vi "Scatter Page.vi"() -> ()   [LabVIEW 2020, in "3D Scatter.lvclass"]
uses:
  <vilib>/Math Plots/3D Math Plots/3D Scatter/3D Scatter/3D Scatter.lvclass
  <vilib>/Math Plots/3D Math Plots/3D Scatter/3D Scatter/Typedef/3D Scatter Property Array.ctl
  <vilib>/Math Plots/3D Math Plots/3D Scatter/3D Scatter/Typedef/3D Scatter Property.ctl
  <vilib>/Math Plots/3D Math Plots/3D Plot/3D Plot/Typedef/Sprite Type.ctl
  <vilib>/Math Plots/3D Math Plots/3D Plot/3D Plot/Typedef/Color Ramp Cluster.ctl
  <vilib>/Math Plots/3D Math Plots/3D Plot/3D Plot/Typedef/Dialog State.ctl
  <vilib>/Math Plots/3D Math Plots/3D Plot/3D Plot/Typedef/Temp Scene State.ctl
  <vilib>/Math Plots/3D Math Plots/3D Plot/3D Plot/Typedef/Temp Scene Property Action.ctl
  <vilib>/Math Plots/3D Math Plots/3D Plot/3D Plot/3D Plot.lvclass
panel:
  in  "Point Size":sgl=0.001 caption="Point size" min=0.001 step=1
  in  "Point Style":u16(ring) caption="Point style"
  out "Scatter Property Out":T1
  in  "Scatter Property In":T1
  out "Color Ramp":dbl[][](graph)
  in  "Color Map Style":u16(ring) caption="Color map style" items=["None ", "Shaded", "Color spectrum", "Grey scale", "Custom"]
  in  "YZ Plane Projection":bool caption="YZ plane projection"
  in  "XZ Plane Projection":bool caption="XZ plane projection"
  in  "XY Plane Projection":bool caption="XY plane projection"
  in  "Coordinate System":u16(ring) caption="Coordinate system" items=["Cartesian", "Cylindrical", "Spherical"]
  in  "Plot Opacity":sgl(slide) caption="Plot opacity(%)" min=0 max=100 scale=0.0..100.0
  in  "Plot List":i32(listbox)
  in  "Ramp Edit":bool caption="Ramp edit"
  in  "Move Down":bool
  in  "Move Up":bool
  in  "Delete":bool
  in  "New":bool
  in  "Event Registration":refnum<event-registration>
  # "Scatter"
  # "General"
  # "Projection"
  # "Color Ramp"
  # "Scatter"
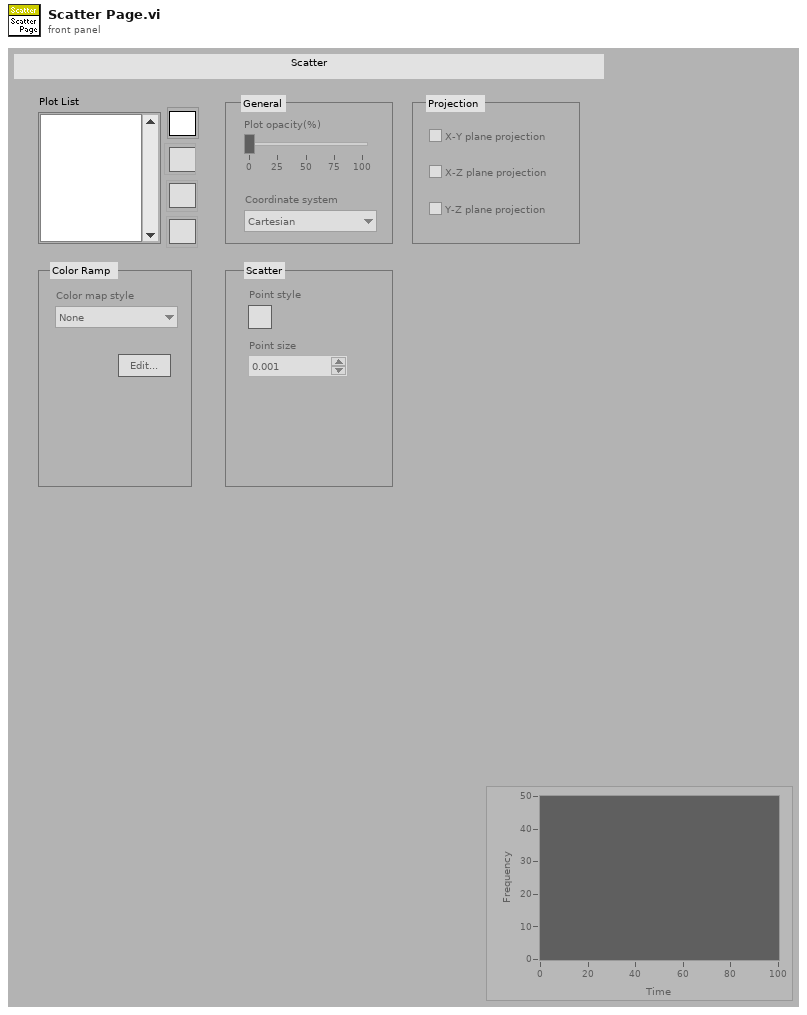
[diagram p1: front panel]
types:
  T1 = typedef "3D Scatter.lvclass/3D Scatter Property Array.ctl" = T2[]
  T2 = typedef "3D Scatter.lvclass/3D Scatter Property.ctl" = cluster{"General Property":cluster{"Plot Name":string, "Coordinate System":enum16{"Cartesian", "Cylindrical", "Spherical"}, "Opacity":sgl}, "Projection Property":cluster{"Draw XY":bool, "Draw YZ":bool, "Draw XZ":bool}, "Plot Property":cluster{"Sprite Type":T3, "Point Size":sgl, "Color Ramp Cluster":T4}}
  T3 = typedef "3D Plot.lvclass/Sprite Type.ctl" = enum16{"None", "Empty Square", "Solid Square", "Empty Diamond", "Solid Diamond", "Empty Circle", "Solid Circle", "Asterisk", "Bold X", "Wireframe Sphere", "Solid Sphere", "Wireframe Cube", "Solid Cube"}
  T4 = typedef "3D Plot.lvclass/Color Ramp Cluster.ctl" = cluster{"Color Ramp Style":enum16{"None", "Shaded", "Color spectrum", "Grey scale", "Custom"}, "Color Ramp Array":u32[], "Color Ramp Index":i32[], "Interpolate?":bool, "Logarithm?":bool}
  T5 = typedef "3D Plot.lvclass/Dialog State.ctl" = enum16{"Initialize", "Read Porperty", "Write Property", "Idle", "Exit"}
  T6 = typedef "3D Plot.lvclass/Temp Scene State.ctl" = enum16{"Create", "Update Scene", "Get Plot Representation", "Destory"}
  T7 = typedef "3D Plot.lvclass/Temp Scene Property Action.ctl" = enum16{"Graph Property", "Light Property", "Axis Property", "Value Pair Property", "Format Property", "Cursor Property", "Plot Specific Property"}
  T8 = typedef "3D Plot.lvclass/Multiplot Representation.ctl" = cluster{"Plot Represention Array":T9[], "Max Range":T10}
  T9 = typedef "3D Plot.lvclass/Plot Representation.ctl" = cluster{"Plot ID":i32, "Plot Range":T10, "Mesh Data":T11, "Dimension":cluster{"X Dimension":i32, "Y Dimension":i32}, "Ramp Range":T10}
  T10 = typedef "3D Plot.lvclass/Range Clusters.ctl" = cluster{"X Range":cluster{"Max X":sgl, "Min X":sgl}, "Y Range":cluster{"Max Y":sgl, "Min Y":sgl}, "Z Range":cluster{"Max Z":sgl, "Min Z":sgl}}
  T11 = typedef "3D Plot.lvclass/Mesh Data.ctl" = cluster{"Index Array":u32[], "Vertex Array":cluster{"X":sgl, "Y":sgl, "Z":sgl}[], "Normal Array":cluster{"X":sgl, "Y":sgl, "Z":sgl}[], "Color Index Array":i32[]}
  T12 = enum16{"None", "Shaded", "Color spectrum", "Grey scale", "Custom"}
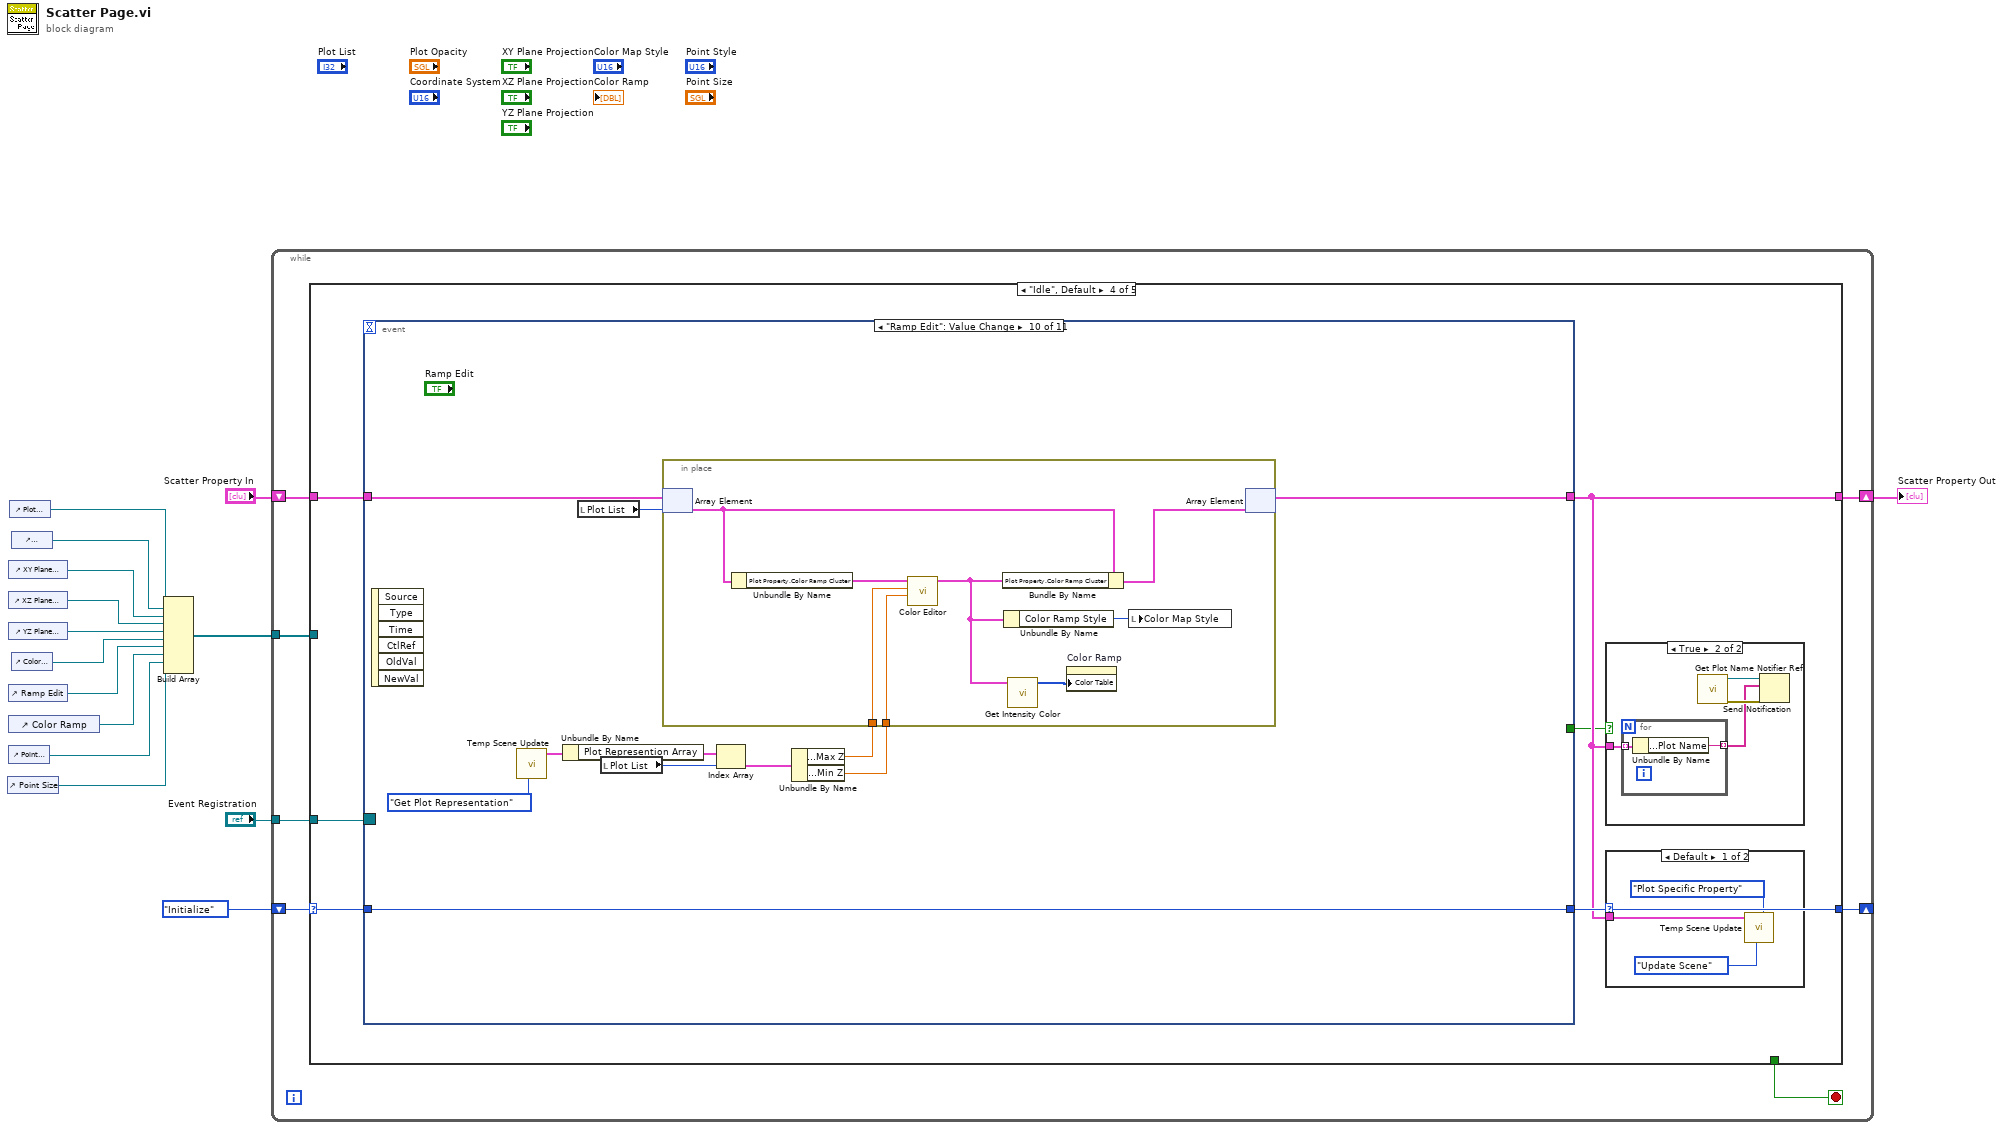
[diagram p0: block diagram]
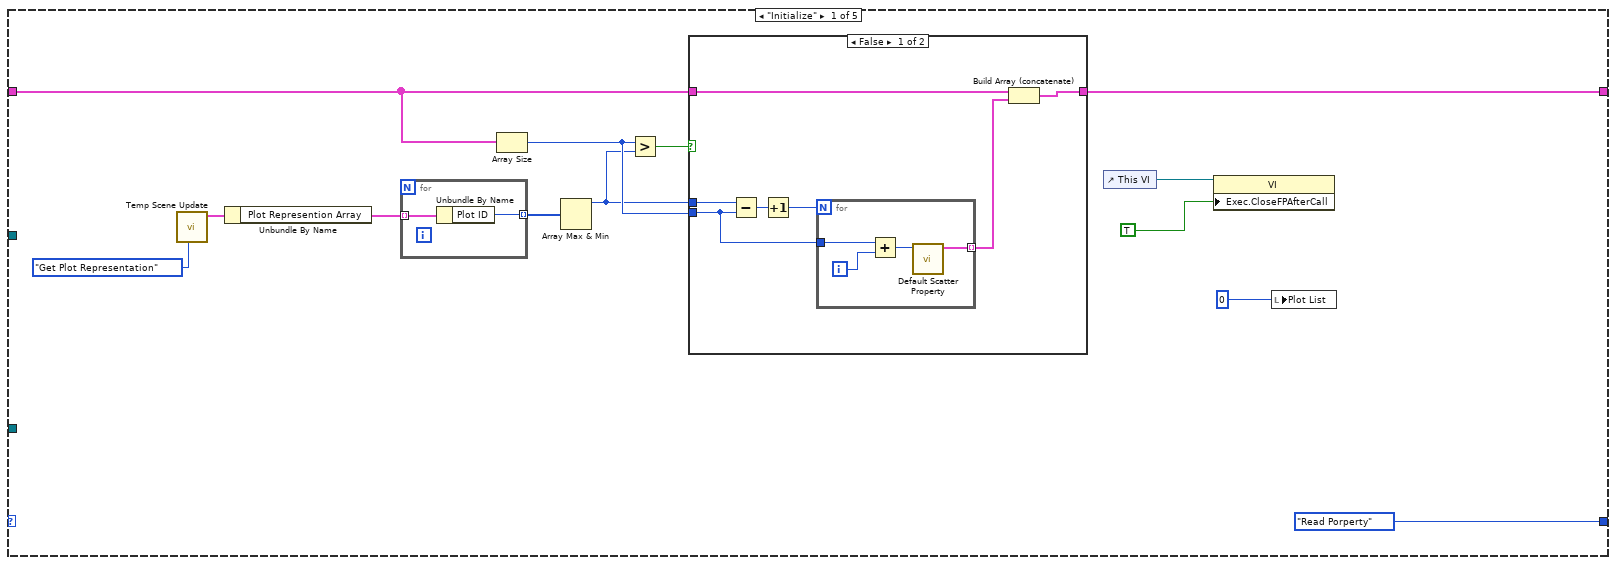
[diagram p2: hidden frame]
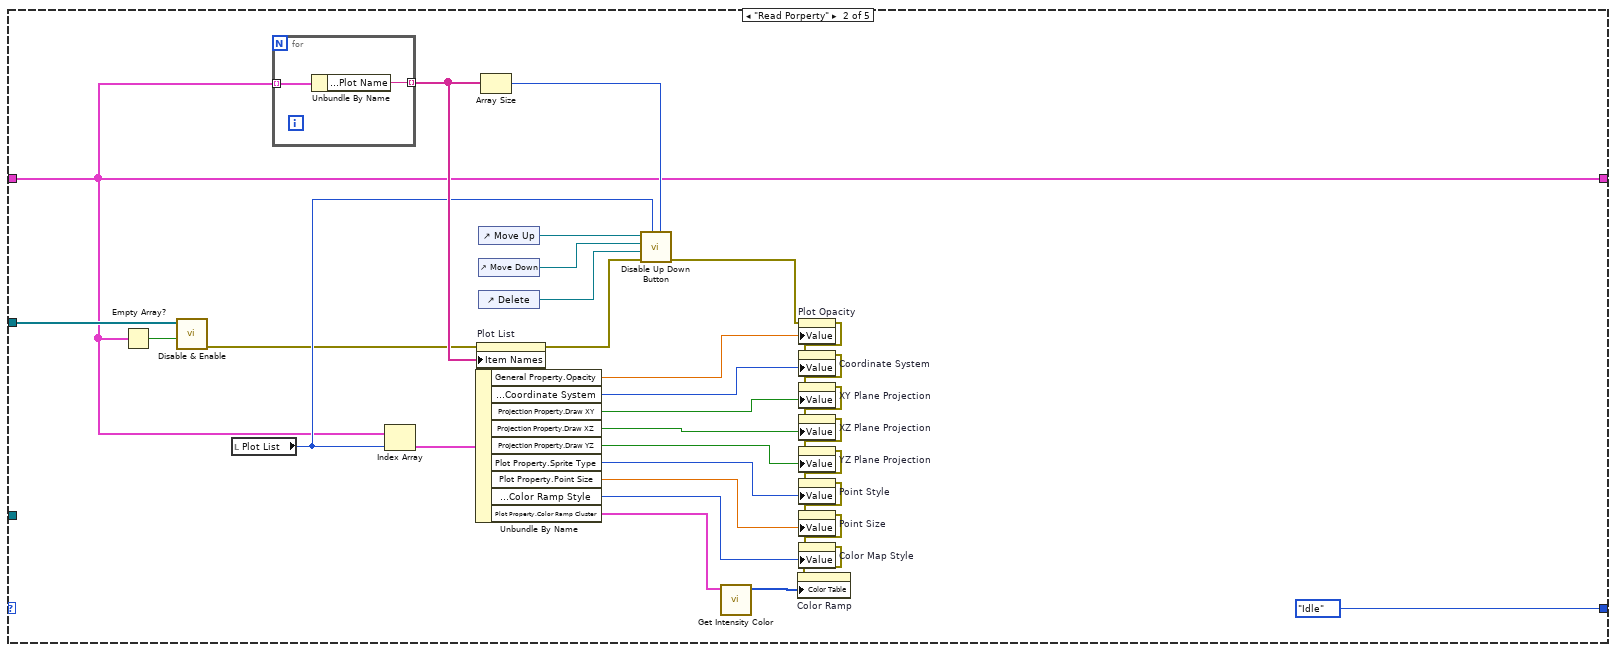
[diagram p4: hidden frame]
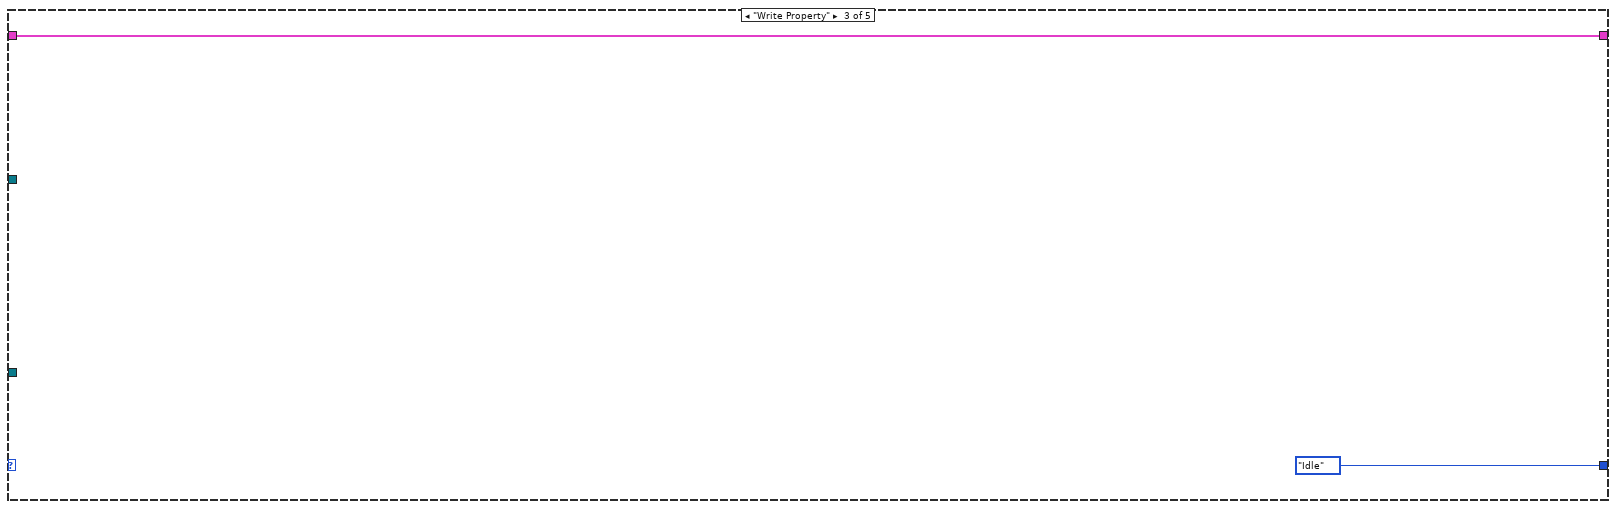
[diagram p5: hidden frame]
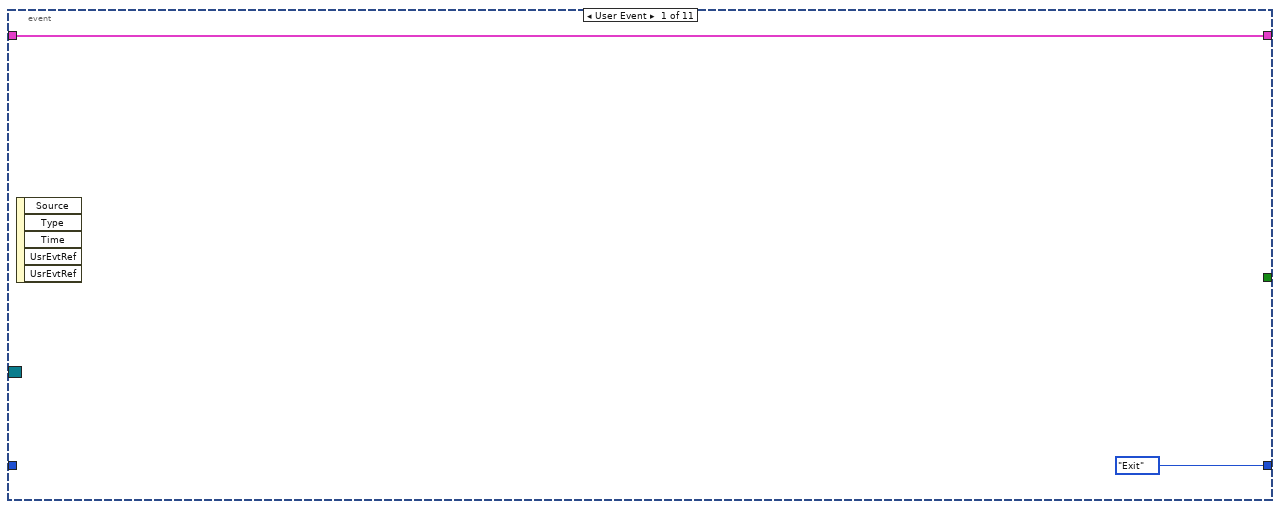
[diagram p8: hidden frame]
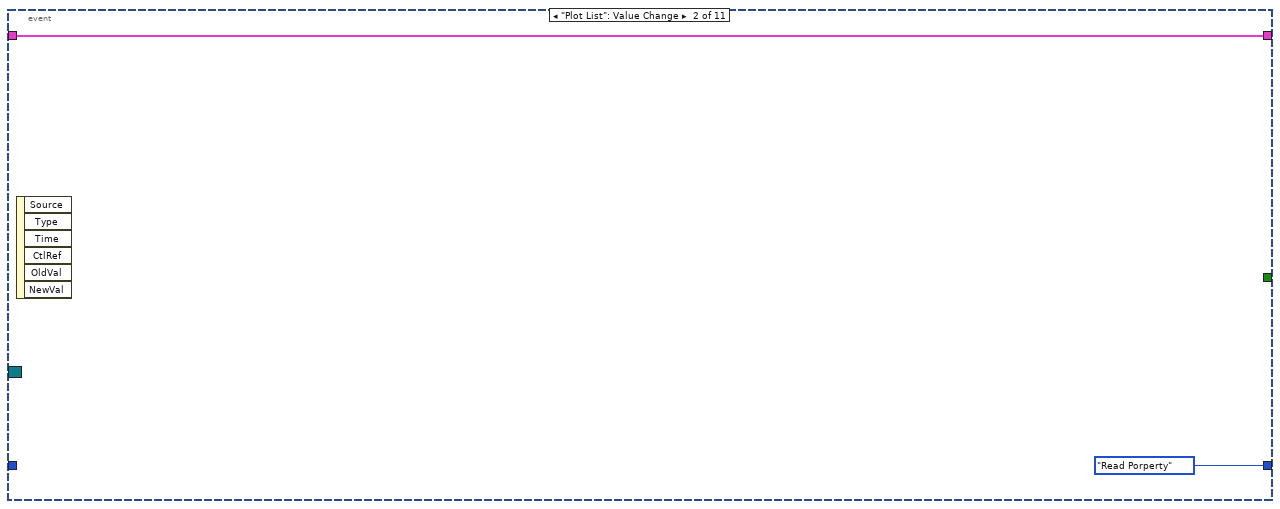
[diagram p9: hidden frame]
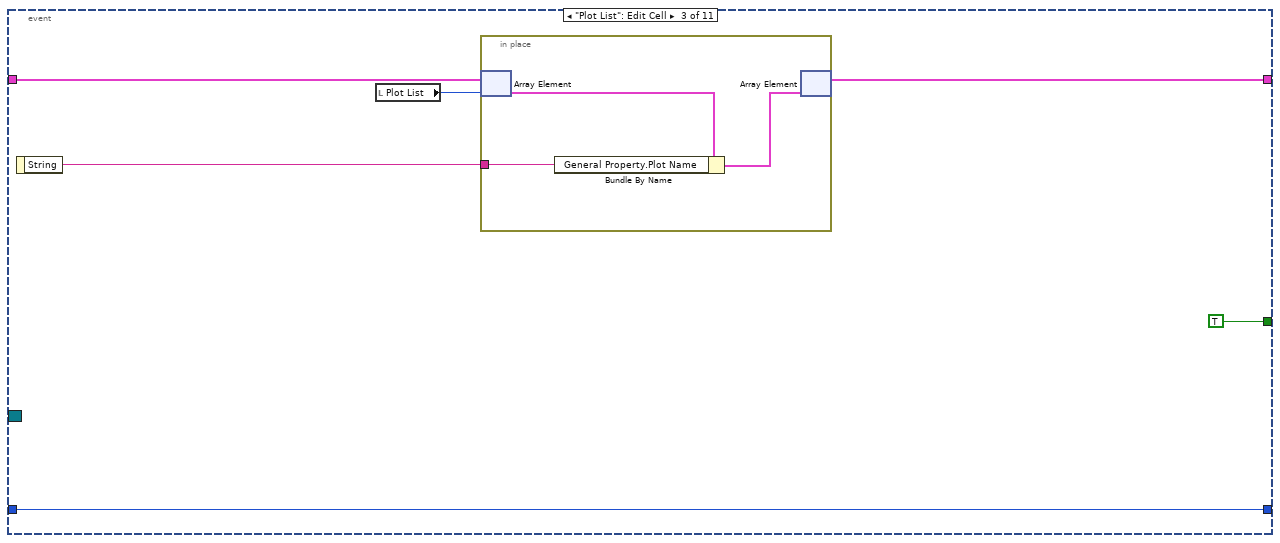
[diagram p10: hidden frame]
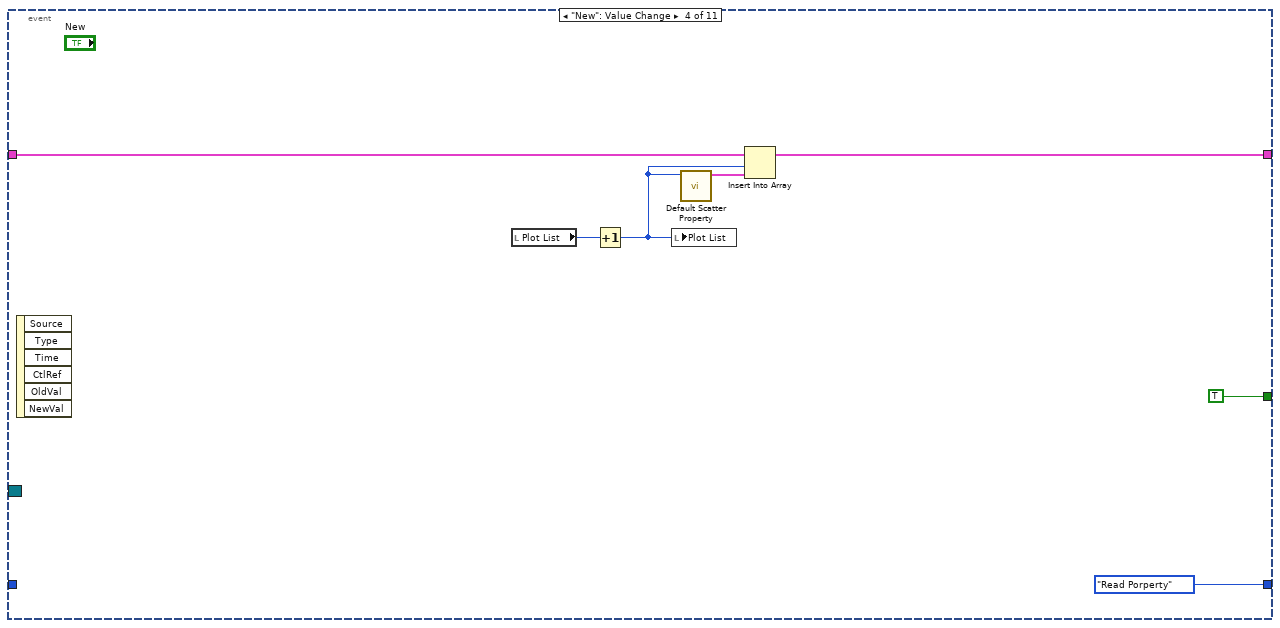
[diagram p11: hidden frame]
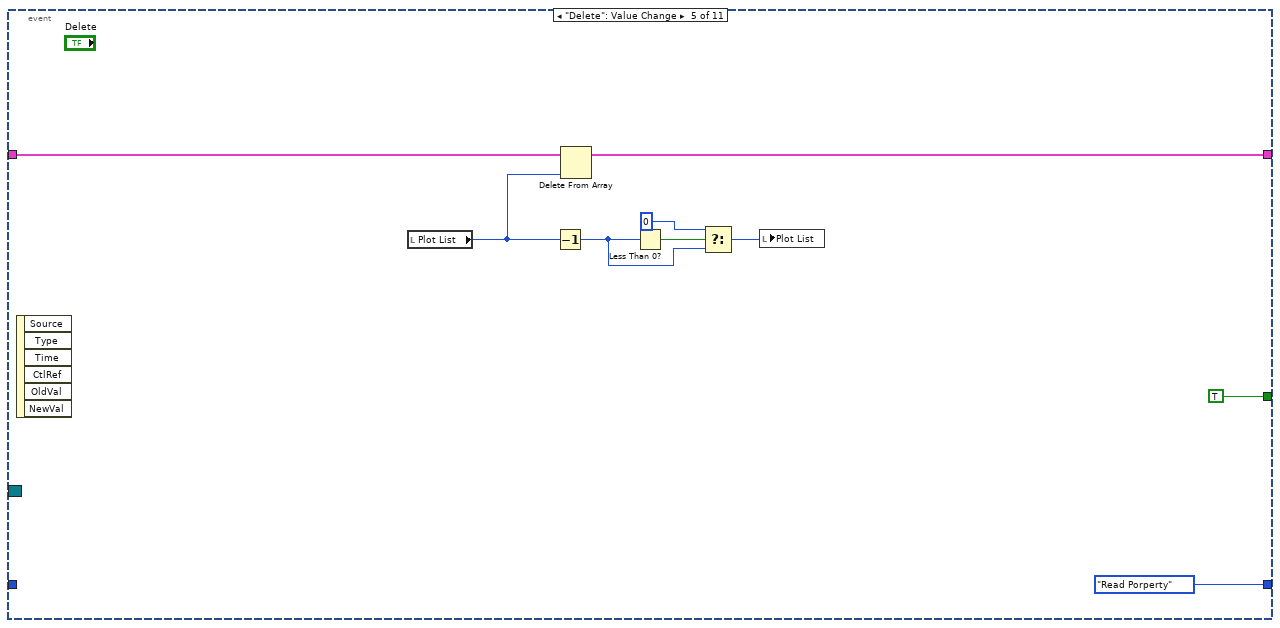
[diagram p12: hidden frame]
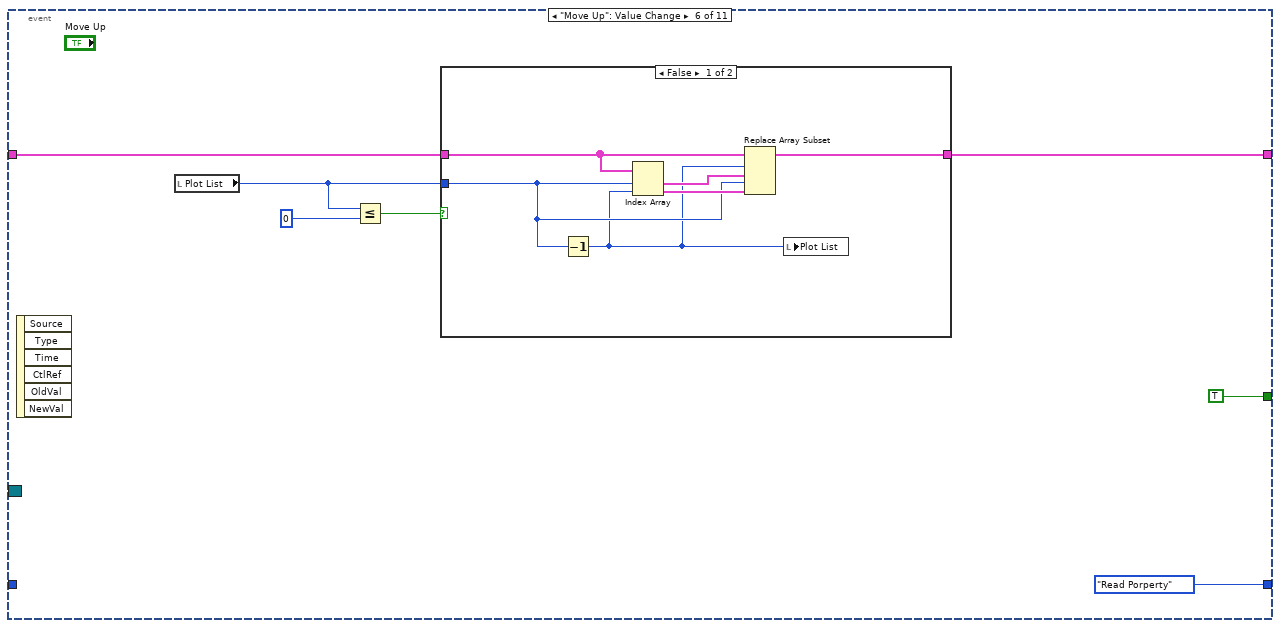
[diagram p13: hidden frame]
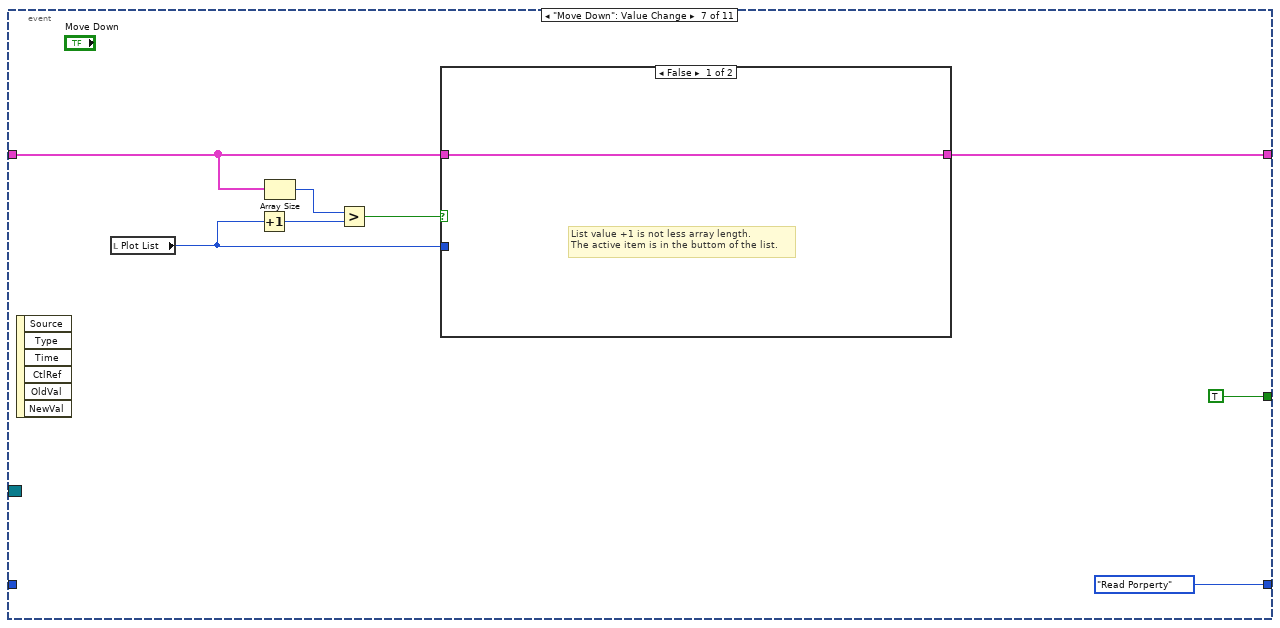
[diagram p15: hidden frame]
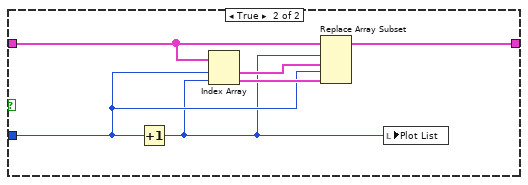
[diagram p16: hidden frame]
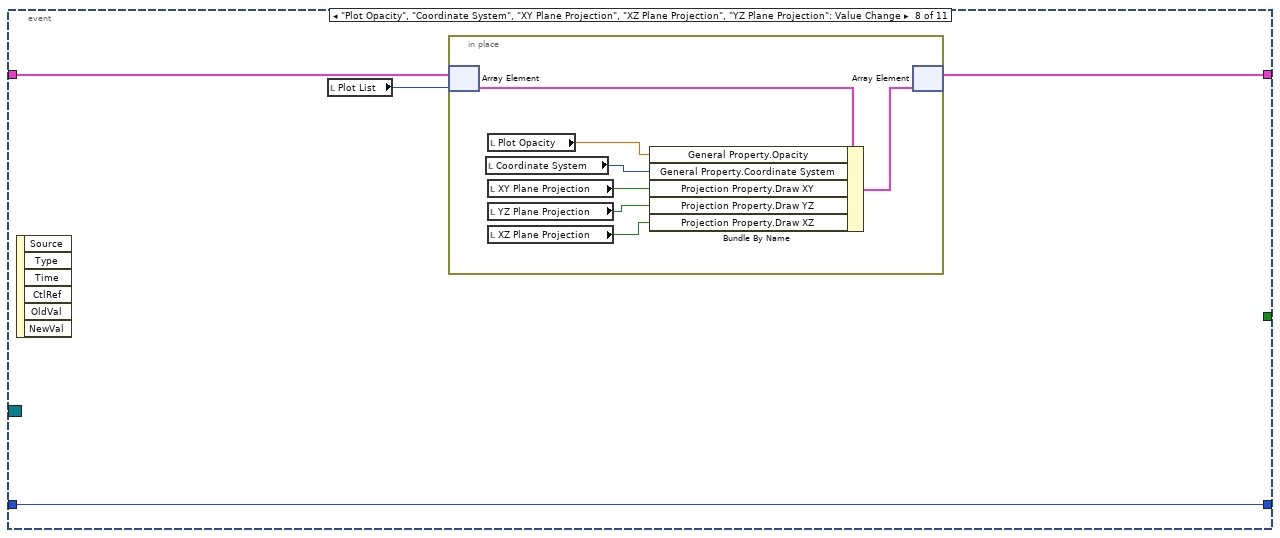
[diagram p17: hidden frame]
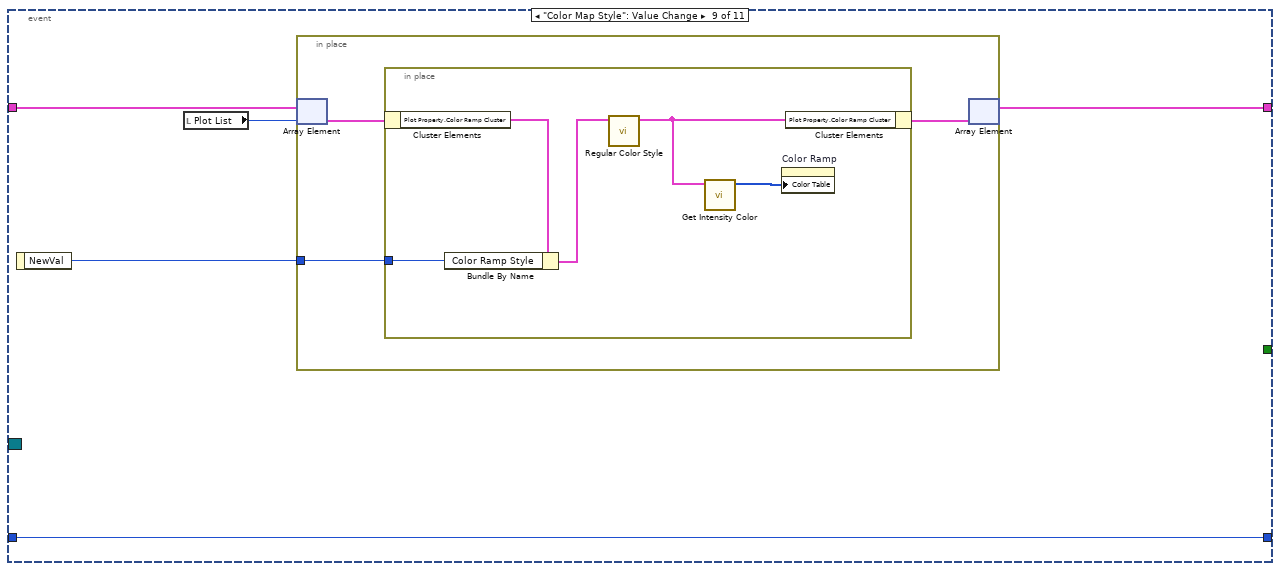
[diagram p18: hidden frame]
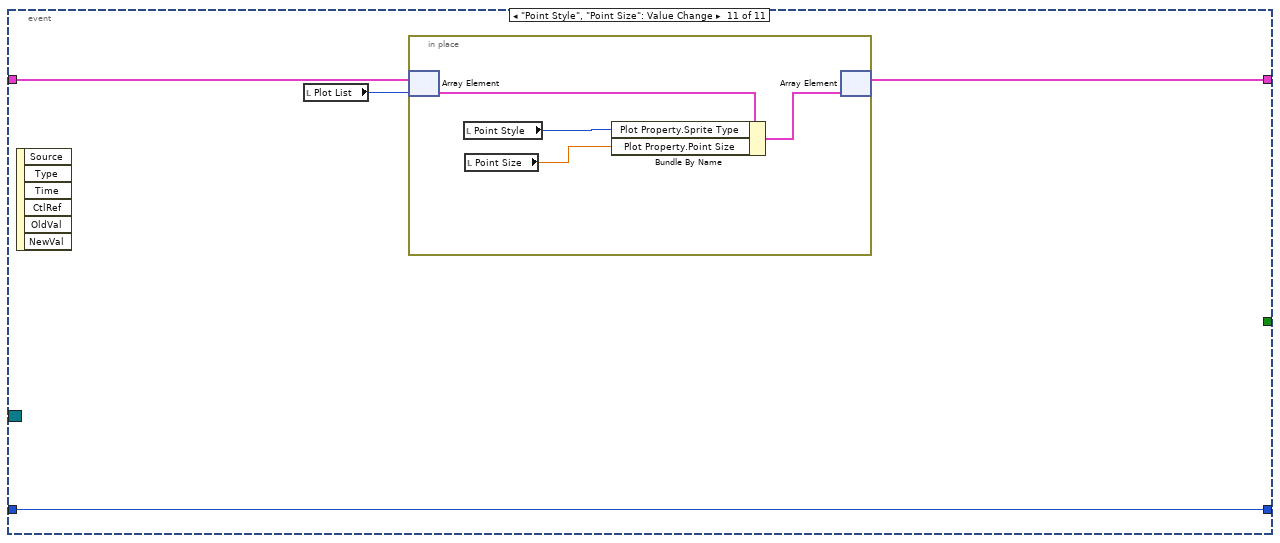
[diagram p19: hidden frame]
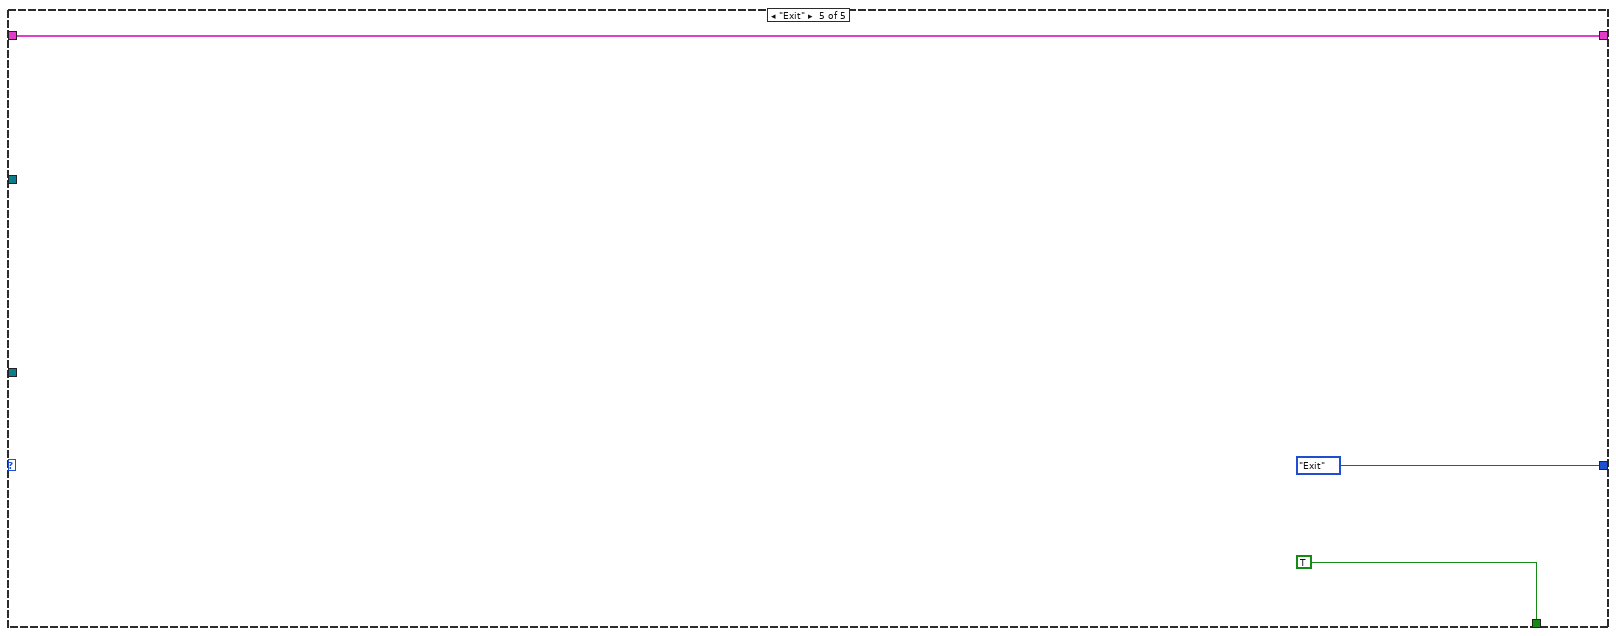
[diagram p20: hidden frame]
diagram:
  n1 = control-ref of="Point Size"() -> (w2:refnum<vi>)
  n2 = control-ref of="XY Plane Projection"() -> (w9:refnum<vi>)
  n3 = control-ref of="XZ Plane Projection"() -> (w8:refnum<vi>)
  n4 = control-ref of="YZ Plane Projection"() -> (w7:refnum<vi>)
  n5 = control-ref of="Ramp Edit"() -> (w5:refnum<vi>)
  n6 = control-ref of="Color Ramp"() -> (w4:refnum<vi>)
  n7 = control-ref of="Point Style"() -> (w3:refnum<vi>)
  n8 = control-ref of="Plot Opacity"() -> (w11:refnum<vi>)
  n9 = control-ref of="Coordinate System"() -> (w10:refnum<vi>)
  n10 = control-ref of="Color Map Style"() -> (w6:refnum<vi>)
  n11 = Build Array(w11, w10, w9, w8, w7, w6, w5, w4, w3, w2) -> (w1:refnum<vi>[])
  n12 = while {
    shift-right: [w21] -> w12
    shift-left: "Scatter Property In" -> [w22]
    shift-right: [w17] -> _
    shift-left: Dialog_State."Initialize" -> [w20]
    tunnel: "Event Registration" -> [w18]
    tunnel: w1 -> [w16]
    stop <- w19 stop-if-true
    n13 = case shown="\"Idle\", Default" w20 {
      selector: w20 -> [_ _ _ w89 _]
      tunnel: w22 -> [w25 w68 w84 w91 w210]
      tunnel: [w24 w68 w84 w87 w210] -> w21
      tunnel: [Dialog_State."Read Porperty" Dialog_State."Idle" Dialog_State."Idle" w88 Dialog_State."Exit"] -> w17
      tunnel: [_ _ _ _ TRUE] -> w19
      tunnel: w18 -> [_ _ _ w90 _]
      tunnel: w16 -> [_ w69 _ _ _]
      frame "Initialize" {
        n14 = call <vilib>:"Temp Scene Update.vi"("State"=Temp_Scene_State."Get Plot Representation") -> ("Multiplot Representation"=w30:T8)  [unwired: 5 in, 5 out]
        n15 = Unbundle By Name(w30) -> ("Plot Represention Array"=w23:T9[])
        n16 = for {
          tunnel: w23 -> [w49] mode=indexing
          tunnel: [w48] -> w29 mode=indexing
          n17 = Unbundle By Name(w49) -> ("Plot ID"=w48:i32)
        }
        n18 = Array Size(array=w25) -> (size(s)=w27:i32)
        n19 = Array Max & Min(array=w29) -> (max value=w26:i32)  [unwired: 3 out]
        n20 = Greater?(x=w27, y=w26) -> (0:w28:bool)
        n21 = case shown="False" w28 {
          tunnel: [w40 w47] -> w24
          tunnel: w25 -> [w42 w47]
          tunnel: w27 -> [w36 _]
          tunnel: w26 -> [w37 _]
          frame False {
            n22 = Subtract(x=w37, y=w36) -> (x-y=w39:i32)
            n23 = Increment(x=w39) -> (x+1=w38:i32)
            n24 = for {
              N: w38 -> [_]
              tunnel: w36 -> [w45]
              tunnel: [w43] -> w41 mode=indexing
              i -> [w46]
              n25 = Add(x=w45, y=w46) -> (x+y=w44:i32)
              n26 = call <vilib>:"Default Scatter Property.vi"("Plot ID"=w44) -> ("Default Property"=w43:T2)  [unwired: 10 out]
            }
            n27 = Build Array (concatenate)(w42, w41) -> (w40:T1)
          }
          frame True {
          }
        }
        n28 = control-ref of="This VI"() -> (w34:refnum<vi>)
        n29 = property class="VI"(reference=w34, "Exec.CloseFPAfterCall"=TRUE ("Execution:Close After Call")) -> ()  [unwired: 1 in, 2 out]
        n30 = local write "Plot List"(0 ("Plot List")) -> ()
      }
      frame "Read Porperty" {
        n31 = Empty Array?(array=w68) -> (empty?=w70:bool)
        n32 = call <vilib>:"Disable & Enable.vi"("Disabled?"=w70, "Control Ref Array"=w69) -> ("error out"=w67:errorcluster)  [unwired: 1 in, 8 out]
        n33 = local read "Plot List"() -> (w71:i32)
        n34 = for {
          tunnel: w68 -> [w83] mode=indexing
          tunnel: [w82] -> w73 mode=indexing
          n35 = Unbundle By Name(w83) -> ("General Property.Plot Name"=w82:string)
        }
        n36 = Index Array(array=w68, index=w71) -> (element=w80:T2)
        n37 = Unbundle By Name(w80) -> ("General Property.Opacity"=w59:sgl, "General Property.Coordinate System"=w58:enum16{"Cartesian", "Cylindrical", "Spherical"}, "Projection Property.Draw XY"=w57:bool, "Projection Property.Draw XZ"=w56:bool, "Projection Property.Draw YZ"=w55:bool, "Plot Property.Sprite Type"=w54:T3, "Plot Property.Point Size"=w53:sgl, "Plot Property.Color Ramp Cluster.Color Ramp Style"=w52:T12, "Plot Property.Color Ramp Cluster"=w79:T4)
        n38 = property on="Plot List" class="LstBox (strict)"(error in=w67, "Item Names"=w73) -> (error out=w72:errorcluster)  [unwired: 1 in, 1 out]
        n39 = control-ref of="Move Up"() -> (w75:refnum<vi>)
        n40 = control-ref of="Move Down"() -> (w76:refnum<vi>)
        n41 = control-ref of="Delete"() -> (w77:refnum<vi>)
        n42 = Array Size(array=w73) -> (size(s)=w74:i32)
        n43 = call <vilib>:"Disable Up Down Button.vi"("Length"=w74, "Index"=w71, "error in (no error)"=w72, "Delete Ref"=w77, "Move Down Ref"=w76, "Move Up Ref"=w75) -> ("error out"=w50:errorcluster)  [unwired: 5 out]
        n44 = call <vilib>:"Get Intensity Color.vi"("Color Ramp Cluster"=w79) -> ("Intensity Color"=w78:u32[])  [unwired: 4 in, 6 out]
        n45 = property on="Plot Opacity" class="Slide (strict)"(error in=w50, "Value"=w59) -> (error out=w66:errorcluster)  [unwired: 1 in, 1 out]
        n46 = property on="Coordinate System" class="Ring (strict)"(error in=w66, "Value"=w58) -> (error out=w65:errorcluster)  [unwired: 1 in, 1 out]
        n47 = property on="XY Plane Projection" class="Bool (strict)"(error in=w65, "Value"=w57) -> (error out=w64:errorcluster)  [unwired: 1 in, 1 out]
        n48 = property on="XZ Plane Projection" class="Bool (strict)"(error in=w64, "Value"=w56) -> (error out=w63:errorcluster)  [unwired: 1 in, 1 out]
        n49 = property on="YZ Plane Projection" class="Bool (strict)"(error in=w63, "Value"=w55) -> (error out=w62:errorcluster)  [unwired: 1 in, 1 out]
        n50 = property on="Point Style" class="Ring (strict)"(error in=w62, "Value"=w54) -> (error out=w61:errorcluster)  [unwired: 1 in, 1 out]
        n51 = property on="Point Size" class="DigNum (strict)"(error in=w61, "Value"=w53) -> (error out=w60:errorcluster)  [unwired: 1 in, 1 out]
        n52 = property on="Color Map Style" class="Ring (strict)"(error in=w60, "Value"=w52) -> (error out=w51:errorcluster)  [unwired: 1 in, 1 out]
        n53 = property on="Color Ramp" class="IntGraph (strict)"(error in=w51, "Color Table"=w78) -> ()  [unwired: 1 in, 2 out]
      }
      frame "Write Property" {
      }
      frame "Idle", Default {
        n54 = event shown="[9] \"Ramp Edit\": Value Change" {
          selector: w90 -> [_ _ _ _ _ _ _ _ _ _ _]
          dyn-events: _ -> [_ _ _ _ _ _ _ _ _ _ _]
          timeout: _ -> [_ _ _ _ _ _ _ _ _ _ _]
          tunnel: w91 -> [w102 w104 w108 w118 w127 w132 w146 w160 w173 w191 w203]
          tunnel: [w102 w104 w107 w117 w128 w131 w145 w159 w170 w190 w202] -> w87
          tunnel: [Dialog_State."Exit" Dialog_State."Read Porperty" w106 Dialog_State."Read Porperty" Dialog_State."Read Porperty" Dialog_State."Read Porperty" Dialog_State."Read Porperty" w162 w174 w193 w204] -> w88
          tunnel: w89 -> [_ _ w106 _ _ _ _ w162 w174 w193 w204]
          tunnel: [_ _ TRUE TRUE TRUE TRUE TRUE _ _ _ _] -> w86
          event User Event {
            n55 = event-data() -> ()  [unwired: 6 out]
          }
          event "Plot List": Value Change {
            n56 = event-data() -> ()  [unwired: 7 out]
          }
          event "Plot List": Edit Cell {
            n57 = event-data() -> ("String"=w109:string)  [unwired: 1 out]
            n58 = local read "Plot List"() -> (w110:i32)
            n59 = in-place {
              in-place-border: w109 -> [w111]
              n60 = in-place-array #1(w108, w110) -> (w113:T2)
              n61 = Bundle By Name(cluster=w113, "General Property.Plot Name"=w111) -> (w112:T2)
              n62 = in-place-array #1(w112) -> (w107:T1)  [unwired: 1 out]
            }
          }
          event "New": Value Change {
            n63 = event-data() -> ()  [unwired: 7 out]
            n64 = local read "Plot List"() -> (w119:i32)
            n65 = Increment(x=w119) -> (x+1=w115:i32)
            n66 = local write "Plot List"(w115) -> ()
            n67 = call <vilib>:"Default Scatter Property.vi"("Plot ID"=w115) -> ("Default Property"=w114:T2)  [unwired: 10 out]
            n68 = Insert Into Array(array=w118, index=w115, new element=w114) -> (w117:T1)
          }
          event "Delete": Value Change {
            n69 = event-data() -> ()  [unwired: 7 out]
            n70 = local read "Plot List"() -> (w123:i32)
            n71 = Decrement(x=w123) -> (x-1=w124:i32)
            n72 = Delete From Array(array=w127, index=w123) -> (array with subset deleted=w128:T1)  [unwired: 1 in, 1 out]
            n73 = Less Than 0?(x=w124) -> (x < 0?=w126:bool)
            n74 = Select(t=0, s=w126, f=w124) -> (s? t:f=w122:i32)
            n75 = local write "Plot List"(w122) -> ()
          }
          event "Move Up": Value Change {
            n76 = event-data() -> ()  [unwired: 7 out]
            n77 = local read "Plot List"() -> (w133:i32)
            n78 = Less Or Equal?(x=w133, y=0) -> (x <= y?=w134:bool)
            n79 = case shown="False" w134 {
              tunnel: w132 -> [w140 w143]
              tunnel: [w139 w143] -> w131
              tunnel: w133 -> [w138 _]
              frame False {
                n80 = Decrement(x=w138) -> (x-1=w137:i32)
                n81 = Index Array(array=w140, index #1=w138, index #2=w137) -> (element #1=w142:T2, element #2=w141:T2)
                n82 = Replace Array Subset(array=w140, new element #1=w142, index #1=w137, new element #2=w141, index #2=w138) -> (w139:T1)
                n83 = local write "Plot List"(w137) -> ()
              }
              frame True {
                # "List value is less or equal to 0.\nThe active item is in the top of the list."
              }
            }
          }
          event "Move Down": Value Change {
            n84 = event-data() -> ()  [unwired: 7 out]
            n85 = local read "Plot List"() -> (w147:i32)
            n86 = Increment(x=w147) -> (x+1=w149:i32)
            n87 = Array Size(array=w146) -> (size(s)=w150:i32)
            n88 = Greater?(x=w150, y=w149) -> (0:w148:bool)
            n89 = case shown="False" w148 {
              tunnel: w146 -> [w152 w156]
              tunnel: [w152 w155] -> w145
              tunnel: w147 -> [_ w154]
              frame False {
                # "List value +1 is not less array length.\nThe active item is in the buttom of the list."
              }
              frame True {
                n90 = Increment(x=w154) -> (x+1=w153:i32)
                n91 = Index Array(array=w156, index #1=w154, index #2=w153) -> (element #1=w158:T2, element #2=w157:T2)
                n92 = Replace Array Subset(array=w156, new element #1=w158, index #1=w153, new element #2=w157, index #2=w154) -> (w155:T1)
                n93 = local write "Plot List"(w153) -> ()
              }
            }
          }
          event "Plot Opacity", "Coordinate System", "XY Plane Projection", "XZ Plane Projection", "YZ Plane Projection": Value Change {
            n94 = event-data() -> ()  [unwired: 7 out]
            n95 = local read "Plot List"() -> (w161:i32)
            n96 = in-place {
              n97 = in-place-array #2(w160, w161) -> (w165:T2)
              n98 = local read "Coordinate System"() -> (w163:u16)
              n99 = local read "Plot Opacity"() -> (w169:sgl)
              n100 = local read "XY Plane Projection"() -> (w168:bool)
              n101 = local read "YZ Plane Projection"() -> (w166:bool)
              n102 = local read "XZ Plane Projection"() -> (w167:bool)
              n103 = Bundle By Name(cluster=w165, "General Property.Opacity"=w169, "General Property.Coordinate System"=w163, "Projection Property.Draw XY"=w168, "Projection Property.Draw YZ"=w166, "Projection Property.Draw XZ"=w167) -> (w164:T2)
              n104 = in-place-array #2(w164) -> (w159:T1)  [unwired: 1 out]
            }
          }
          event "Color Map Style": Value Change {
            n105 = event-data() -> ("NewVal"=w171:u16)  [unwired: 1 out]
            n106 = local read "Plot List"() -> (w172:i32)
            n107 = in-place {
              in-place-border: w171 -> [w176]
              n108 = in-place-array #3(w173, w172) -> (w177:T2)
              n109 = in-place {
                in-place-border: w176 -> [w181]
                n110 = in-place-cluster #4(w177) -> ("Plot Property.Color Ramp Cluster"=w182:T4)
                n111 = Bundle By Name(cluster=w182, "Color Ramp Style"=w181) -> (w180:T4)
                n112 = call <vilib>:"Regular Color Style.vi"("Color Ramp Cluster in"=w180) -> ("Color Ramp Cluster out"=w178:T4)  [unwired: 10 in]
                n113 = call <vilib>:"Get Intensity Color.vi"("Color Ramp Cluster"=w178) -> ("Intensity Color"=w179:u32[])  [unwired: 4 in, 6 out]
                n114 = property on="Color Ramp" class="IntGraph (strict)"("Color Table"=w179) -> ()  [unwired: 2 in, 2 out]
                n115 = in-place-cluster #4("Plot Property.Color Ramp Cluster"=w178) -> (w175:T2)
              }
              n116 = in-place-array #3(w175) -> (w170:T1)  [unwired: 1 out]
            }
          }
          event "Ramp Edit": Value Change {
            n117 = event-data() -> ()  [unwired: 7 out]
            n118 = call <vilib>:"Temp Scene Update.vi"("State"=Temp_Scene_State."Get Plot Representation") -> ("Multiplot Representation"=w186:T8)  [unwired: 5 in, 5 out]
            n119 = Unbundle By Name(w186) -> ("Plot Represention Array"=w183:T9[])
            n120 = local read "Plot List"() -> (w192:i32)
            n121 = local read "Plot List"() -> (w189:i32)
            n122 = Index Array(array=w183, index=w189) -> (element=w188:T9)
            n123 = Unbundle By Name(w188) -> ("Plot Range.Z Range.Max Z"=w185:sgl, "Plot Range.Z Range.Min Z"=w184:sgl)
            n124 = in-place {
              in-place-border: w185 -> [w195]
              in-place-border: w184 -> [w194]
              n125 = in-place-array #5(w191, w192) -> (w200:T2)
              n126 = Unbundle By Name(w200) -> ("Plot Property.Color Ramp Cluster"=w199:T4)
              n127 = call <vilib>:"Color Editor.vi"("Min"=w194, "Max"=w195, "Color Ramp Cluster in"=w199) -> ("Color Ramp Cluster out"=w197:T4)  [unwired: 3 in, 5 out]
              n128 = Bundle By Name(cluster=w200, "Plot Property.Color Ramp Cluster"=w197) -> (w201:T2)
              n129 = Unbundle By Name(w197) -> ("Color Ramp Style"=w196:T12)
              n130 = call <vilib>:"Get Intensity Color.vi"("Color Ramp Cluster"=w197) -> ("Intensity Color"=w198:u32[])  [unwired: 4 in, 6 out]
              n131 = property on="Color Ramp" class="IntGraph (strict)"("Color Table"=w198) -> ()  [unwired: 2 in, 2 out]
              n132 = local write "Color Map Style"(w196) -> ()
              n133 = in-place-array #5(w201) -> (w190:T1)  [unwired: 1 out]
            }
          }
          event "Point Style", "Point Size": Value Change {
            n134 = event-data() -> ()  [unwired: 7 out]
            n135 = local read "Plot List"() -> (w205:i32)
            n136 = in-place {
              n137 = in-place-array #6(w203, w205) -> (w209:T2)
              n138 = local read "Point Style"() -> (w206:u16)
              n139 = local read "Point Size"() -> (w207:sgl)
              n140 = Bundle By Name(cluster=w209, "Plot Property.Sprite Type"=w206, "Plot Property.Point Size"=w207) -> (w208:T2)
              n141 = in-place-array #6(w208) -> (w202:T1)  [unwired: 1 out]
            }
          }
        }
        n142 = case shown="True" w86 {
          tunnel: w87 -> [_ w92]
          frame False {
          }
          frame True {
            n143 = for {
              tunnel: w92 -> [w97] mode=indexing
              tunnel: [w96] -> w93 mode=indexing
              n144 = Unbundle By Name(w97) -> ("General Property.Plot Name"=w96:string)
            }
            n145 = call <vilib>:"Get Plot Name Notifier Ref.vi"() -> ("error out"=w95:errorcluster, "Plot Names Notifier Ref"=w94:refnum<notifier>)  [unwired: 1 in, 9 out]
            n146 = Send Notification(notification=w93, notifier=w94, error in (no error)=w95) -> ()  [unwired: 2 out]
          }
        }
        n147 = case shown="Default" w88 {
          tunnel: w87 -> [w100 _]
          frame Default {
            n148 = call <vilib>:"Temp Scene Update.vi"("Property Name"=Temp_Scene_Property_Action."Plot Specific Property", "State"=Temp_Scene_State."Update Scene", "Property In"=w100) -> ()  [unwired: 3 in, 6 out]
          }
          frame "Exit" {
          }
        }
      }
      frame "Exit" {
      }
    }
  }
  "Scatter Property Out" <- w12
